vi "Write Binary Revovery File.vi"(8 "error in (no error)":errorcluster, 10 "Data In":dbl[](array[numeric]), 11 "Path":path) -> (0 "error out":errorcluster)   [LabVIEW 2015]
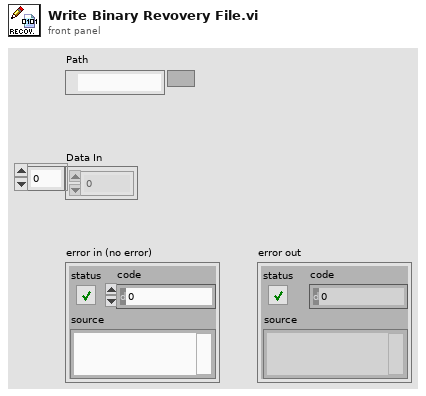
[diagram p1: front panel]
types:
  T1 = enum16{"open", "replace", "create", "open or create", "replace or create", "replace or create with confirmation"}
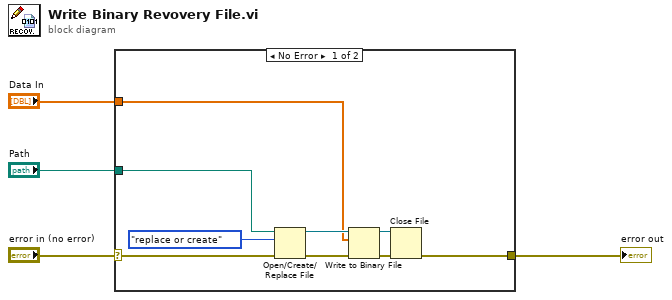
[diagram p0: block diagram]
diagram:
  n1 = case shown="No Error" "error in (no error)" {
    selector: "error in (no error)" -> [w11 w14]
    tunnel: [w13 w14] -> w3
    tunnel: "Path" -> [w12 _]
    tunnel: "Data In" -> [w6 _]
    frame No Error {
      n2 = Open/Create/Replace File(file path (use dialog)=w12, error in=w11, operation (0:open)=T1."replace or create") -> (refnum out=w10:refnum<file>, error out=w9:errorcluster)  [unwired: 3 in, 1 out]
      n3 = Write to Binary File(file (use dialog)=w10, data=w6, error in=w9) -> (refnum out=w8:refnum<file>, error out=w7:errorcluster)  [unwired: 3 in, 1 out]
      n4 = Close File(refnum=w8, error in=w7) -> (error out=w13:errorcluster)  [unwired: 1 out]
    }
    frame Error {
    }
  }
  "error out" <- w3
